vi "Read Msg Q.vi"(8 "error in (no error)":errorcluster, 11 "Msg Q in":refnum<class "Msg Q.lvclass">) -> (0 "error out":errorcluster, 2 "Msg Q":refnum<data-value>, 3 "Msg Q out":refnum<class "Msg Q.lvclass">)   [LabVIEW 2021, in "LVCAM.lvlib" / "Msg Q.lvclass"]
uses:
  Msg Q.lvclass
  Msg/Msg.lvclass
  Msg Q.lvclass/Msg Q.ctl
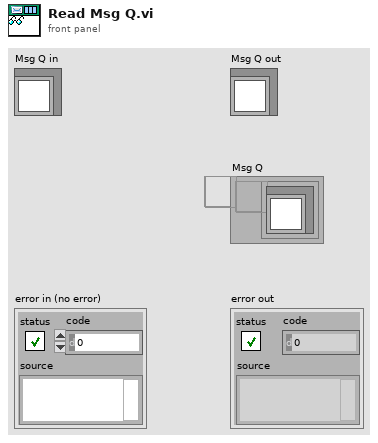
[diagram p1: front panel]
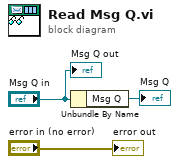
[diagram p0: block diagram]
diagram:
  n1 = Unbundle By Name("Msg Q in") -> ("Msg Q"=→"Msg Q":refnum<data-value>)
  "error out" <- "error in (no error)"
  "Msg Q out" <- "Msg Q in"
